vi "New VI new branch.vi"() -> ()   [LabVIEW 2018]
panel:
  out "Cluster":cluster{"Boolean":bool}
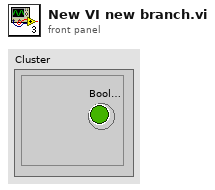
[diagram p1: front panel]
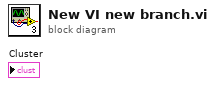
[diagram p0: block diagram]
diagram:
